vi "RealSense_HelloWorld_Left_Right_IR.vi"() -> ()   [LabVIEW 2017]
doc: "This demo shows how to connect a RealSense D4xx Stereo Depth Camera, and stream the LEFT and the RIGHT raw unrectified images."
uses:
  libRealSense3.lvlib
panel:
  out "Output stream format":T1
  in  "laser on/off":bool
  out "Left IR":picture
  out "Right IR":picture
  out "iteration":i32
  in  "stop":bool=TRUE
  out "release frame error":string="No Error"
  out "Capture1 Error":string="No Error"
  out "Config error":string="No Error\rNo Error"
  out "init results":T2={"camera name"="Intel RealSense 415", "camera S/N"="725112060291", "F/W"="05.08.09.00", "Sensor name"="Stereo Module", "api_version"=20710, "rscontext"=659718592, "device_list"=396628960, "device count"=2, "Dev out"=662505184, "sensor_list"=395031584, "sensor count"=2, "Sensor out"=662178704}
  out "init error":string="No Error\rNo Error\rNo Error\rNo Error\rNo Error\rNo Error\rNo Error\rNo Error\rNo Error\rNo Error\rNo Error"
  out "Close Error":string="No Error\rNo Error\rNo Error\rNo Error"
  out "Start Error":string="No Error\rNo Error\rNo Error"
  out "Capture2 error":string="No Error"
  in  "Select Resolution":u16(ring)=3 items=["424 x 240 @6fps", "424 x 240 @15fps", "424 x 240 @30fps", "424 x 240 @60fps", "424 x 240 @90fps", "480 x 270 @6fps", "480 x 270 @15fps", "480 x 270 @30fps", "480 x 270 @60fps", "480 x 270 @90fps", "640 x 360 @6fps", "640 x 360 @15fps", "640 x 360 @30fps", "640 x 360 @60fps", "640 x 360 @90fps", "640 x 480 @6fps", "640 x 480 @15fps", "640 x 480 @30fps", "640 x 480 @60fps", "640 x 480 @90fps", "848 x 480 @6fps", "848 x 480 @15fps", "848 x 480 @30fps", "848 x 480 @60fps", "848 x 480 @90fps", "1280 x 720 @6fps", "1280 x 720 @15fps", "1280 x 720 @30fps", "1280 x 800 @15fps", "1280 x 800 @30fps"]
  # "RealSense Hello World: Left-Right Rectified"
  # "This demo shows how to connect a RealSense D4xx Stereo Depth Camera, and stream the LEFT and the RIGHT images."
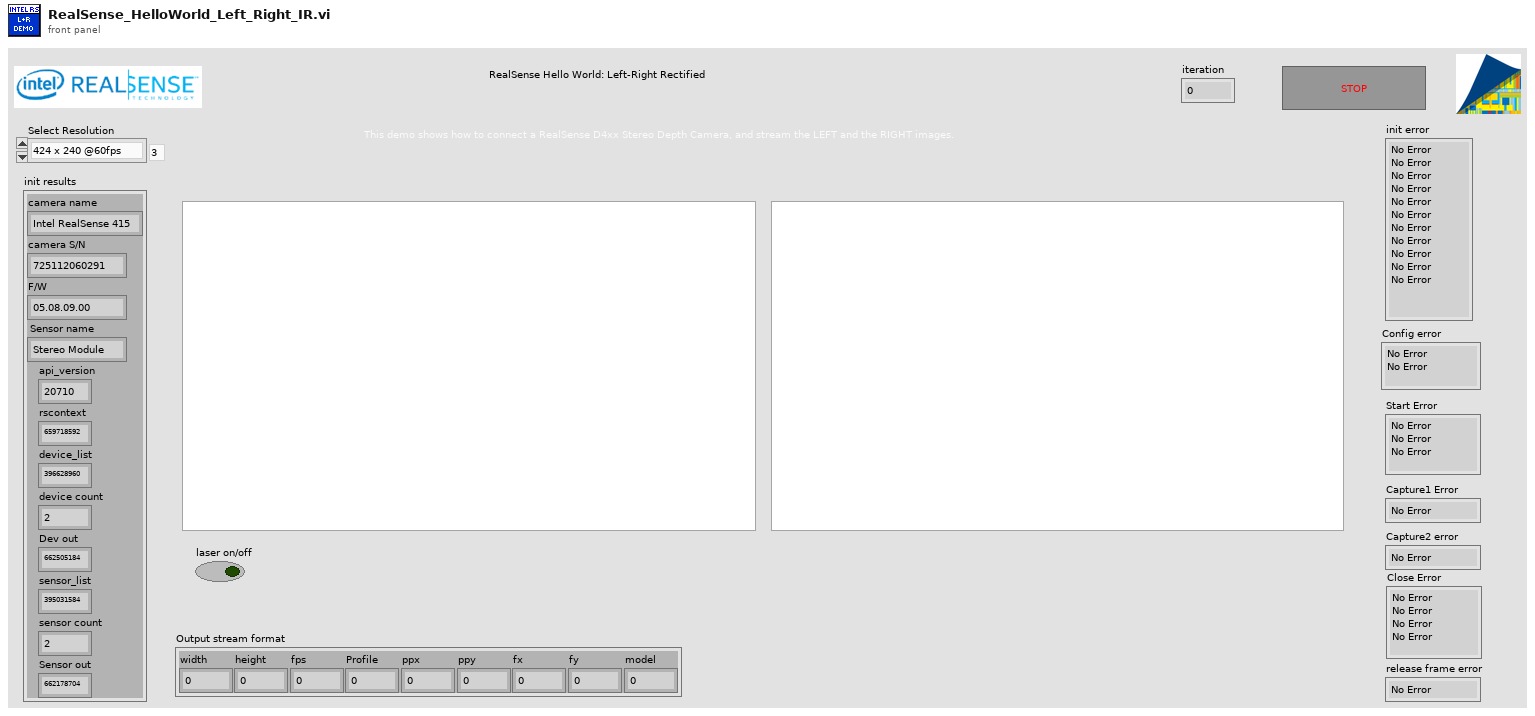
[diagram p1: front panel]
types:
  T1 = cluster{"width":i32, "height":i32, "fps":i32, "Profile":u64, "ppx":sgl, "ppy":sgl, "fx":sgl, "fy":sgl, "model":u32}
  T2 = cluster{"camera name":string, "camera S/N":string, "F/W":string, "Sensor name":string, "api_version":i32, "rscontext":u64, "device_list":u64, "device count":i32, "Dev out":u64, "sensor_list":u64, "sensor count":i32, "Sensor out":u64}
  T3 = enum16{"Depth", "Color (ext.)", "Color (left) ", "IR Left", "IR Right", "IR Left (Y16)", "IR Right (Y16)"}
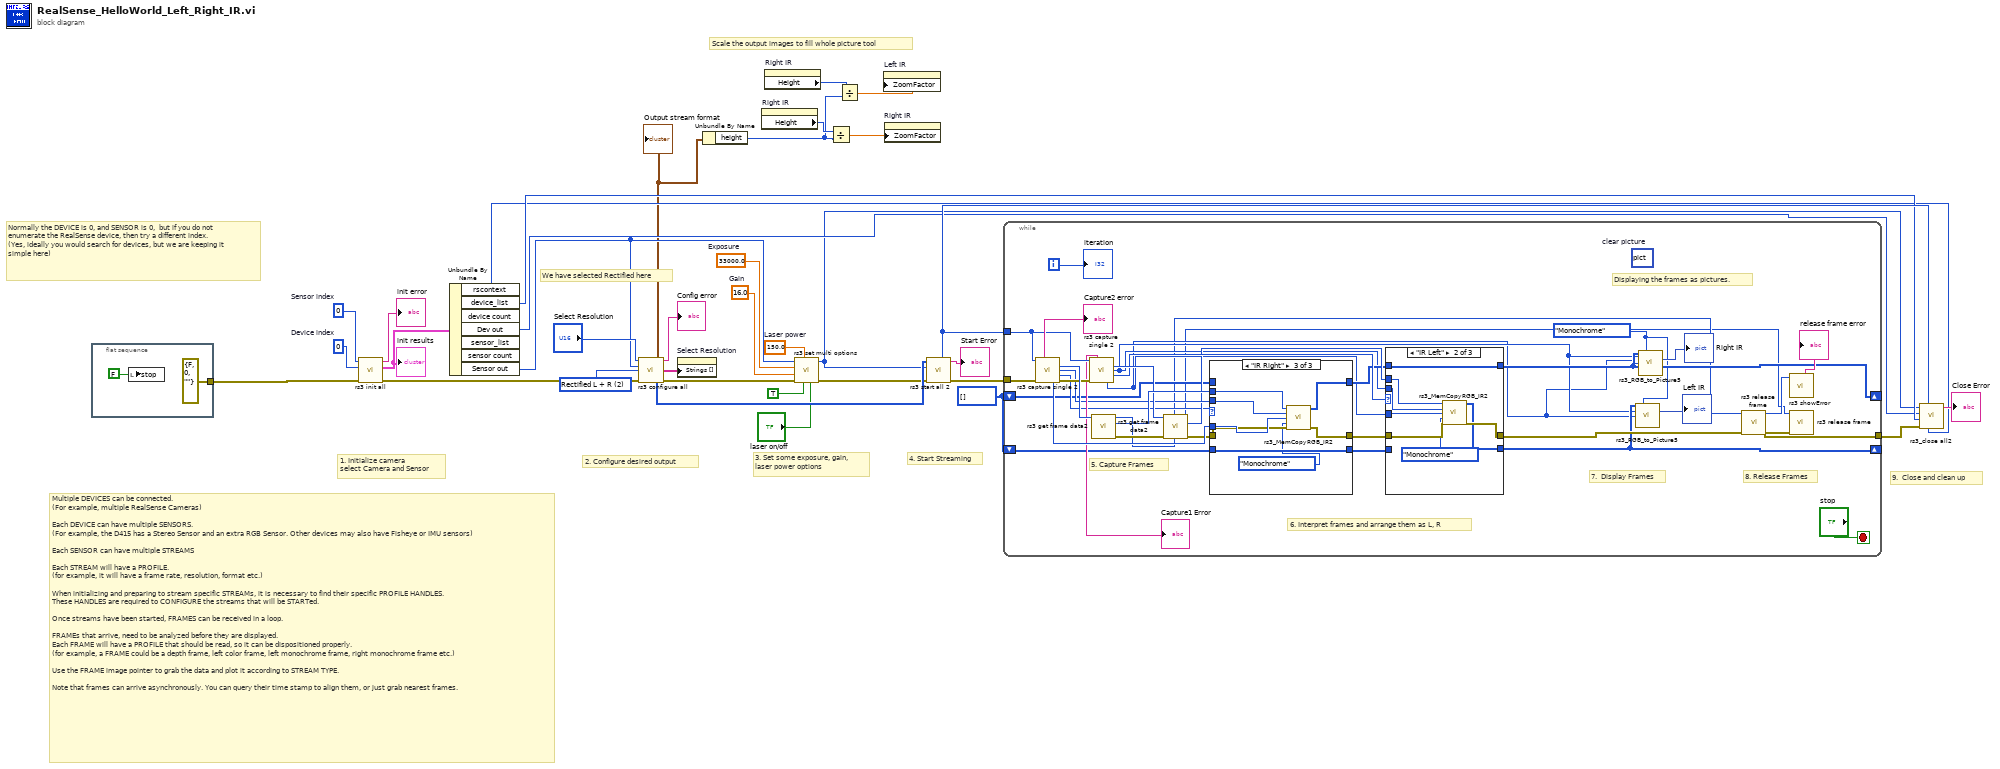
[diagram p0: block diagram]
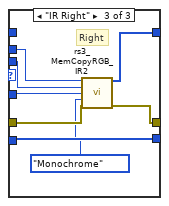
[diagram p3: hidden frame]
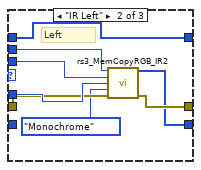
[diagram p5: hidden frame]
diagram:
  w1 = u16 2 items=["Depth + Left Color", "Unrectified L + R", "Rectified L + R", "Depth Only", "RGB ext. Only", "Depth + L Monochrome"] ("Stream selection")
  w9 = u8[] [] ("Output Array")
  w35 = 0  # Device index
  w34 = 0  # Sensor index
  w11 = sgl 16.0  # Gain
  w12 = sgl 150.0  # Laser power
  w13 = sgl 33000.0  # Exposure
  # "Scale the output images to fill whole picture tool"
  # "We have selected Rectified here"
  # "Normally the DEVICE is 0, and SENSOR is 0,  but if you do not enumerate the RealSense device, then try a different index.\n(Yes, ideally you would search for devices, but we are keeping it simple here)"
  # "Multiple DEVICES can be connected. \n(For example, multiple RealSense Cameras)\n\nEach DEVICE can have multiple SENSORS. \n(For example, the D415 has a Stereo Sensor and an extra RGB Sensor. Other devices may also have Fisheye or IMU sensors) \n\nEach SENSOR can have multiple STREAMS\n\nEach STREAM will have a PROFILE. \n(for example, it will have a frame rate, resolution, format etc.)\n\nWhen initializing and preparing to stream specific STREAMs, it is necessary to find their specific PROFILE HANDLES.\nThese HANDLES are required to CONFIGURE the streams that will be STARTed. \n\nOnce streams have been started, FRAMES can be received in a loop. \n \nFRAMEs that arrive, need to be analyzed before they are displayed. \nEach FRAME will have a PROFILE that should be read, so it can be dispositioned properly.\n(for example, a FRAME could be a depth frame, left color frame, left monochrome frame, right monochrome frame etc.)\n\nUse the FRAME image pointer to grab the data and plot it according to STREAM TYPE.\n\nNote that frames can arrive asynchronously. You can query their time stamp to align them, or just grab nearest frames."
  # "9.  Close and clean up"
  # "4. Start Streaming"
  # "3. Set some exposure, gain, \nlaser power options"
  # "2. Configure desired output"
  # "1. Initialize camera\nselect Camera and Sensor"
  n1 = flat-sequence {
    tunnel: [errorcluster {"status"=FALSE, "code"=0, "source"=""} ("error in")] -> w18
    frame #0 {
      n2 = local write "stop"(FALSE ("stop")) -> ()
    }
  }
  n3 = call "rs3 init all.vi"("error in"=w18, "Select Device"=w35, "Select Sensor"=w34) -> ("error out"=w33:errorcluster, "init results"=w26:T2, "init error"=→"init error":string)  [unwired: 2 in, 4 out]
  "init results" <- w26
  n4 = Unbundle By Name(w26) -> ("rscontext"=w24:u64, "device_list"=w25:u64, "Dev out"=w21:u64, "Sensor out"=w15:u64)  [unwired: 3 out]
  n5 = call "rs3 configure all.vi"("Select Resolution"="Select Resolution", "Sensor in"=w15, "Stream selection"=w1, "error in (no error)"=w33) -> ("Output stream L"=w7:T1, "config error"=→"Config error":string, "Output stream"=w19:string[], "Stream Profile Handles"=w32:u64[], "error out"=w17:errorcluster)  [unwired: 2 in, 5 out]
  "Output stream format" <- w7
  n6 = property on="Select Resolution" class="Ring (strict)"("Strings []"=w19) -> ()  [unwired: 2 in, 2 out]
  n7 = Unbundle By Name(w7) -> ("height"=w4:i32)
  n8 = property on="Right IR" class="Pict"() -> ("Height"=w6:u32)  [unwired: 2 in, 2 out]
  n9 = property on="Right IR" class="Pict"() -> ("Height"=w3:u32)  [unwired: 2 in, 2 out]
  n10 = call "rs3 set multi options.vi"("laser on/off"="laser on/off", "autoexposure"=TRUE, "Laser power, mW (0-360)"=w12, "error in (no error)"=w17, "Gain(16-248)"=w11, "Exposure, us"=w13, "Sensor in"=w15) -> ("error out"=w16:errorcluster, "Sensor out"=w14:u64)  [unwired: 2 in, 1 out]
  n11 = Divide(x=w6, y=w4) -> (x/y=w5:dbl)
  n12 = Divide(x=w3, y=w4) -> (x/y=w2:dbl)
  n13 = property on="Left IR" class="Pict"("ZoomFactor"=w2) -> ()  [unwired: 2 in, 2 out]
  n14 = property on="Right IR" class="Pict"("ZoomFactor"=w5) -> ()  [unwired: 2 in, 2 out]
  n15 = call "rs3 start all 2.vi"("error in (no error)"=w16, "Sensor in"=w14, "Stream profile array"=w32) -> ("error out"=w20:errorcluster, "Config Error"=→"Start Error":string, "queue out"=w31:u64)  [unwired: 5 in, 1 out]
  n16 = while {
    tunnel: w31 -> [w62]
    tunnel: w20 -> [w73]
    tunnel: [w67] -> w30
    shift-right: [w45] -> _
    shift-left: w9 -> [w50]
    shift-right: [w46] -> _
    shift-left: w9 -> [w48]
    i -> [w72]
    stop <- "stop" stop-if-true
    w38 = enum16{"Monochrome", "RGB internal (RGB)"}."Monochrome" ("Color format")
    (unwired) picture bytes[33]  # clear picture
    # "Displaying the frames as pictures."
    # "8. Release Frames"
    # "7.  Display Frames"
    # "6. Interpret frames and arrange them as L, R"
    # "5. Capture Frames"
    n17 = call "rs3 capture single 2.vi"("queue in"=w62, "error in (no error)"=w73) -> ("Capture Error"=→"Capture2 error":string, "frame out"=w71:u64, "width"=w59:i32, "Stream type"=w51:T3, "height"=w69:i32, "error out"=w63:errorcluster)  [unwired: 2 in, 6 out]
    n18 = call "rs3 capture single 2.vi"("queue in"=w62, "error in (no error)"=w63) -> ("Capture Error"=→"Capture1 Error":string, "frame out"=w60:u64, "width"=w44:i32, "Stream type"=w53:T3, "height"=w43:i32)  [unwired: 2 in, 7 out]
    n19 = call "rs3 get frame data2.vi"("frame in"=w71) -> ("error out"=w66:errorcluster, "image pointer out"=w70:u64, "Frame out"=w42:u64)  [unwired: 7 in, 1 out]
    n20 = call "rs3 get frame data2.vi"("error in (no error)"=w66, "frame in"=w60) -> ("error out"=w65:errorcluster, "image pointer out"=w52:u64, "Frame out"=w41:u64)  [unwired: 6 in, 1 out]
    n21 = case shown="\"IR Right\"" w51 {
      tunnel: [w95 w99 w107] -> w55
      tunnel: w70 -> [_ w103 w111]
      tunnel: w59 -> [_ w102 w110]
      tunnel: w69 -> [_ w101 w109]
      tunnel: w65 -> [w95 w100 w108]
      tunnel: [w94 w98 w106] -> w49
      tunnel: w50 -> [w94 _ w106]
      tunnel: w48 -> [w93 w97 _]
      tunnel: [w93 w97 w105] -> w47
      frame "Color (ext.)", Default {
      }
      frame "IR Left" {
        # "Left"
        n22 = call "rs3_MemCopyRGB_IR2.vi"("Zimage pointer"=w103, "RGB  X, width"=w102, "RGB Y, height"=w101, "Color format"=enum16{"Monochrome", "RGB internal (RGB)"}."Monochrome", "error in (no error)"=w100) -> ("Output Array"=w98:u8[], "error out"=w99:errorcluster)  [unwired: 8 in, 1 out]
      }
      frame "IR Right" {
        n23 = call "rs3_MemCopyRGB_IR2.vi"("Zimage pointer"=w111, "RGB  X, width"=w110, "RGB Y, height"=w109, "Color format"=enum16{"Monochrome", "RGB internal (RGB)"}."Monochrome", "error in (no error)"=w108) -> ("Output Array"=w105:u8[], "error out"=w107:errorcluster)  [unwired: 8 in, 1 out]
      }
    }
    n24 = case shown="\"IR Left\"" w53 {
      tunnel: [w76 w82 w89] -> w54
      tunnel: w52 -> [_ w84 w92]
      tunnel: w44 -> [_ w80 w87]
      tunnel: w43 -> [_ w81 w88]
      tunnel: w55 -> [w76 w83 w90]
      tunnel: w49 -> [w74 _ w86]
      tunnel: w47 -> [w75 w79 _]
      tunnel: [w75 w79 w91] -> w46
      tunnel: [w74 w78 w86] -> w45
      frame "Color (ext.)", Default {
      }
      frame "IR Left" {
        n25 = call "rs3_MemCopyRGB_IR2.vi"("Zimage pointer"=w84, "RGB  X, width"=w80, "RGB Y, height"=w81, "Color format"=enum16{"Monochrome", "RGB internal (RGB)"}."Monochrome", "error in (no error)"=w83) -> ("Output Array"=w78:u8[], "error out"=w82:errorcluster)  [unwired: 8 in, 1 out]
      }
      frame "IR Right" {
        # "Right"
        n26 = call "rs3_MemCopyRGB_IR2.vi"("Zimage pointer"=w92, "RGB  X, width"=w87, "RGB Y, height"=w88, "Color format"=enum16{"Monochrome", "RGB internal (RGB)"}."Monochrome", "error in (no error)"=w90) -> ("Output Array"=w91:u8[], "error out"=w89:errorcluster)  [unwired: 8 in, 1 out]
      }
    }
    n27 = call "rs3_RGB_to_Picture5.vi"("RGB array"=w45, "Color format"=w38, "RGB  X, width"=w44, "RGB Y, height"=w43) -> ("new picture"=→"Left IR":picture)  [unwired: 10 in, 1 out]
    n28 = call "rs3_RGB_to_Picture5.vi"("RGB array"=w46, "Color format"=w38, "RGB  X, width"=w44, "RGB Y, height"=w43) -> ("new picture"=→"Right IR":picture)  [unwired: 10 in, 1 out]
    n29 = call "rs3 release frame.vi"("error in (no error)"=w54, "Frame"=w42) -> ("error out"=w68:errorcluster, "error"=w58:u64)  [unwired: 8 in]
    n30 = call "rs3 showError.vi"("error"=w58) -> ("Error summary"=→"release frame error":string)  [unwired: 6 in, 4 out]
    n31 = call "rs3 release frame.vi"("error in (no error)"=w68, "Frame"=w41) -> ("error out"=w67:errorcluster)  [unwired: 8 in, 1 out]
    "iteration" <- w72
  }
  n32 = call "rs3_close all2.vi"("rscontext"=w24, "queue in"=w31, "error in (no error)"=w30, "device_list"=w25, "Dev in"=w21, "Sensor in"=w14) -> ("Close Error"=→"Close Error":string)  [unwired: 4 in, 1 out]
